vi "Task Update Message.vi"(8 "error in (no error)":errorcluster, 10 "Task Update Message":string, 11 "BuildServer in":refnum<class "BuildServer.lvclass">) -> (0 "error out":errorcluster, 3 "BuildServer out":refnum<class "BuildServer.lvclass">)   [LabVIEW 2017, in "BuildServer.lvlib" / "BuildServer.lvclass"]
uses:
  BuildServer.lvclass
  BuildServer.lvclass/BuildServer.ctl
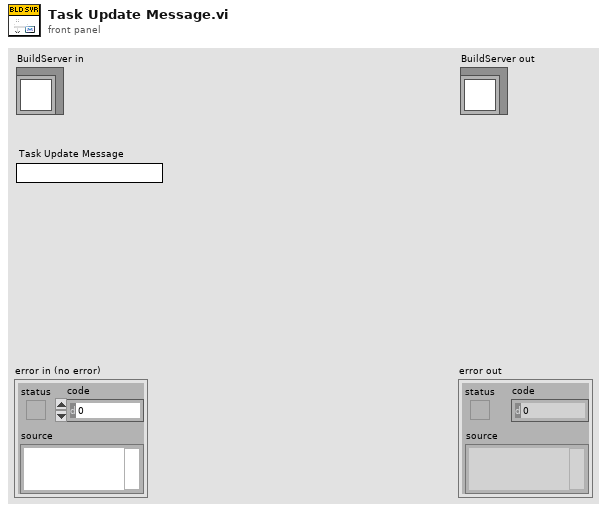
[diagram p1: front panel]
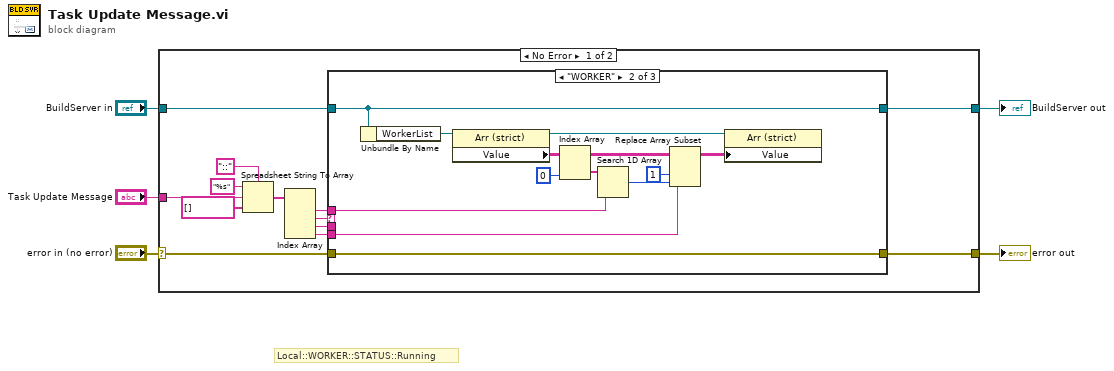
[diagram p0: block diagram]
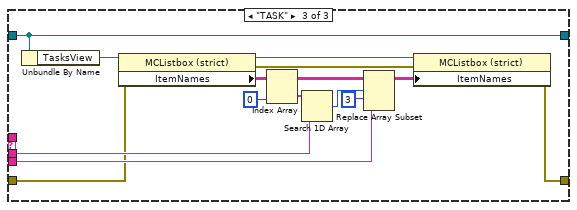
[diagram p3: hidden frame]
diagram:
  # "Local::WORKER::STATUS::Running"
  n1 = case shown="No Error" "error in (no error)" {
    selector: "error in (no error)" -> [w8 w48]
    tunnel: [w7 w48] -> w4
    tunnel: [w9 w47] -> w2
    tunnel: "BuildServer in" -> [w10 w47]
    tunnel: "Task Update Message" -> [w18 _]
    frame No Error {
      n2 = Spreadsheet String To Array(delimiter (Tab)="::", format string="%s", spreadsheet string=w18, array type (2D Dbl)=string[] []) -> (array=w14:string[])
      n3 = Index Array(array=w14) -> (element #1=w6:string, element #2=w13:string, element #3=w12:string, element #4=w11:string)  [unwired: 4 in]
      n4 = case shown="\"WORKER\"" w13 {
        tunnel: w12 -> [_ _ w43]
        tunnel: w11 -> [_ w23 w39]
        tunnel: w10 -> [w20 w31 w46]
        tunnel: [w20 w31 w46] -> w9
        tunnel: w8 -> [w19 w32 w36]
        tunnel: [w19 w32 w34] -> w7
        tunnel: w6 -> [_ w27 _]
        frame Default {
        }
        frame "WORKER" {
          n5 = Unbundle By Name(w31) -> ("WorkerList"=w30:refnum<vi>)
          n6 = property class="Arr (strict)"(reference=w30) -> (reference out=w22:refnum<vi>, "Value"=w26:string[][])  [unwired: 1 in, 1 out]
          n7 = Index Array(array=w26, index (col)=0 ("disabled index (col)")) -> (element=w28:string[])  [unwired: 1 in]
          n8 = Search 1D Array(1D array=w28, element=w27) -> (index of element=w24:i32)  [unwired: 1 in]
          n9 = Replace Array Subset(array=w26, new element=w23, index (row)=w24, index (col)=1 ("disabled index (col)")) -> (w21:string[][])
          n10 = property class="Arr (strict)"(reference=w22, "Value"=w21) -> ()  [unwired: 1 in, 2 out]
        }
        frame "TASK" {
          n11 = Unbundle By Name(w46) -> ("TasksView"=w45:refnum<vi>)
          n12 = property class="MCListbox (strict)"(reference=w45, error in=w36) -> (reference out=w38:refnum<vi>, error out=w35:errorcluster, "ItemNames"=w42:string[][])
          n13 = Index Array(array=w42, index (col)=0 ("disabled index (col)")) -> (element=w44:string[])  [unwired: 1 in]
          n14 = Search 1D Array(1D array=w44, element=w43) -> (index of element=w41:i32)  [unwired: 1 in]
          n15 = Replace Array Subset(array=w42, new element=w39, index (row)=w41, index (col)=3 ("disabled index (col)")) -> (w37:string[][])
          n16 = property class="MCListbox (strict)"(reference=w38, error in=w35, "ItemNames"=w37) -> (error out=w34:errorcluster)  [unwired: 1 out]
        }
      }
    }
    frame Error {
    }
  }
  "error out" <- w4
  "BuildServer out" <- w2
